vi "ArrayTransformations.vi"(10 "?":T1=enum."Transpose", 11 "Input":u32[][](array[numeric])) -> (3 "Transformed Array":u32[][](array[numeric]))   [LabVIEW 2017]
uses:
  Transformation Mode.ctl
panel:
  # "This VI shows how to apply all simple symmetry operations to a 2D array.\n\nChristian Altenbach, altenbach@gmail.com"
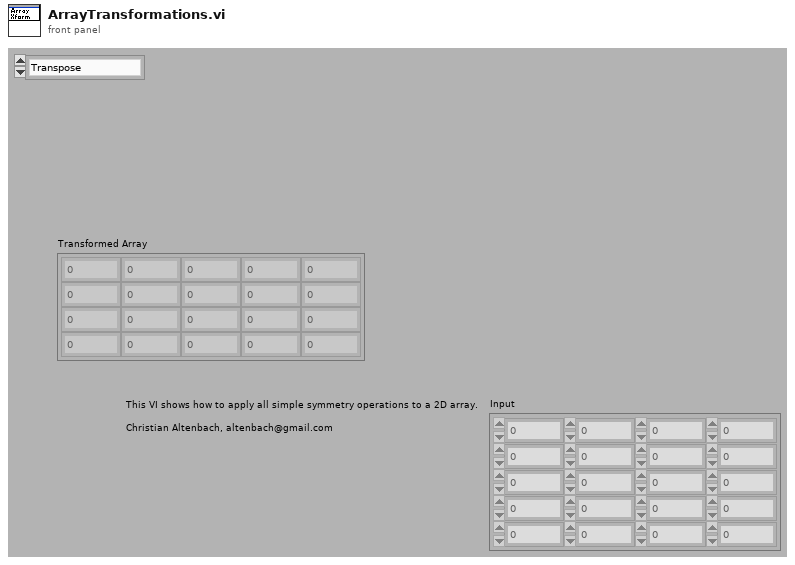
[diagram p1: front panel]
types:
  T1 = typedef "Transformation Mode.ctl" = enum16{"None", "Transpose", "Vertical Flip", "Horizontal Flip", "Rotate 90", "Rotate 270", "Rotate 180", "Diagonal Flip"}
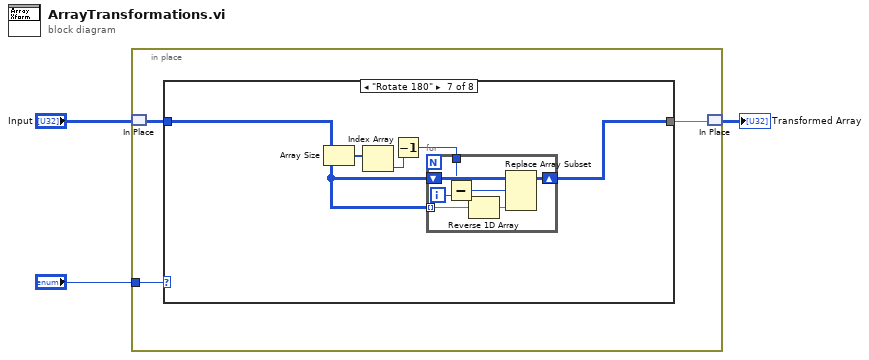
[diagram p0: block diagram]
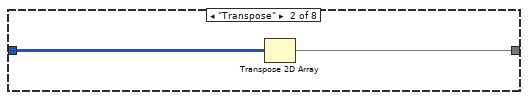
[diagram p3: hidden frame]
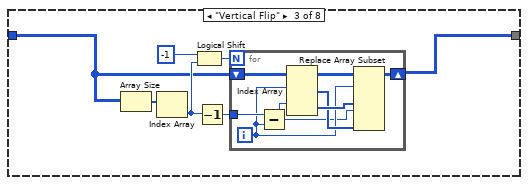
[diagram p4: hidden frame]
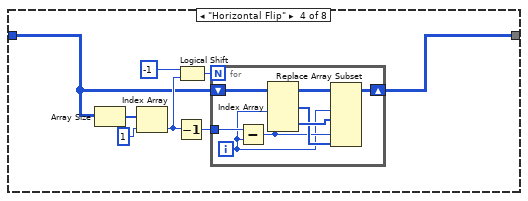
[diagram p5: hidden frame]
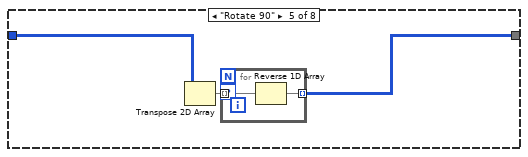
[diagram p6: hidden frame]
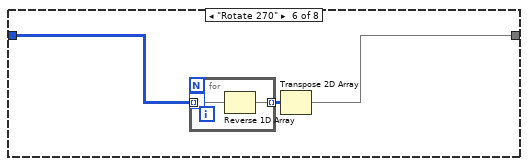
[diagram p7: hidden frame]
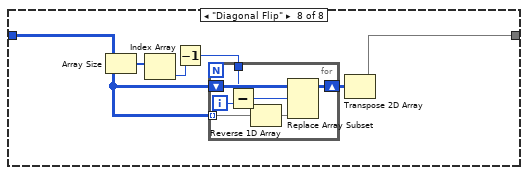
[diagram p8: hidden frame]
diagram:
  n1 = in-place {
    in-place-border: "?" -> [w6]
    n2 = in-place-match #1("Input") -> (w5:u32[][])
    n3 = case shown="\"Rotate 180\"" w6 {
      tunnel: w5 -> [w7 w9 w11 w25 w40 w45 w50 w62]
      tunnel: [w7 w8 w10 w24 w39 w44 w49 w61] -> w4
      frame "None", Default {
      }
      frame "Transpose" {
        n4 = Transpose 2D Array(2D array=w9) -> (transposed array=w8:u32[][])
      }
      frame "Vertical Flip" {
        n5 = Array Size(array=w11) -> (size(s)=w12:i32[])
        n6 = Index Array(array=w12) -> (element=w14:i32)  [unwired: 1 in]
        n7 = Logical Shift(y=i8 -1, x=w14) -> (x << y=w13:i32)
        n8 = Decrement(x=w14) -> (x-1=w16:i32)
        n9 = for {
          N: w13 -> [_]
          shift-right: [w23] -> w10
          shift-left: w11 -> [w22]
          tunnel: w16 -> [w19]
          i -> [w18]
          n10 = Subtract(x=w19, y=w18) -> (x-y=w17:i32)
          n11 = Index Array(array=w22, index (row) #1=w18, index (row) #2=w17) -> (element #1=w20:u32[], element #2=w21:u32[])  [unwired: 2 in]
          n12 = Replace Array Subset(array=w22, new element #1=w21, index (row) #1=w18, new element #2=w20, index (row) #2=w17) -> (w23:u32[][])  [unwired: 2 in]
        }
      }
      frame "Horizontal Flip" {
        n13 = Array Size(array=w25) -> (size(s)=w30:i32[])
        n14 = Index Array(array=w30, index=1) -> (element=w28:i32)
        n15 = Decrement(x=w28) -> (x-1=w26:i32)
        n16 = Logical Shift(y=i8 -1, x=w28) -> (x << y=w29:i32)
        n17 = for {
          N: w29 -> [_]
          shift-right: [w38] -> w24
          shift-left: w25 -> [w37]
          tunnel: w26 -> [w34]
          i -> [w32]
          n18 = Subtract(x=w34, y=w32) -> (x-y=w33:i32)
          n19 = Index Array(array=w37, index (col) #1=w32, index (col) #2=w33) -> (element #1=w35:u32[], element #2=w36:u32[])  [unwired: 2 in]
          n20 = Replace Array Subset(array=w37, new element #1=w36, index (col) #1=w32, new element #2=w35, index (col) #2=w33) -> (w38:u32[][])  [unwired: 2 in]
        }
      }
      frame "Rotate 90" {
        n21 = Transpose 2D Array(2D array=w40) -> (transposed array=w41:u32[][])
        n22 = for {
          tunnel: w41 -> [w43] mode=indexing
          tunnel: [w42] -> w39 mode=indexing
          workers-P: _ -> [_]
          n23 = Reverse 1D Array(array=w43) -> (reversed array=w42:u32[])
        }
      }
      frame "Rotate 270" {
        n24 = for {
          tunnel: w45 -> [w48] mode=indexing
          tunnel: [w47] -> w46 mode=indexing
          workers-P: _ -> [_]
          n25 = Reverse 1D Array(array=w48) -> (reversed array=w47:u32[])
        }
        n26 = Transpose 2D Array(2D array=w46) -> (transposed array=w44:u32[][])
      }
      frame "Rotate 180" {
        n27 = Array Size(array=w50) -> (size(s)=w51:i32[])
        n28 = Index Array(array=w51) -> (element=w53:i32)  [unwired: 1 in]
        n29 = Decrement(x=w53) -> (x-1=w52:i32)
        n30 = for {
          shift-right: [w60] -> w49
          shift-left: w50 -> [w59]
          tunnel: w52 -> [w57]
          tunnel: w50 -> [w54] mode=indexing
          i -> [w58]
          n31 = Subtract(x=w57, y=w58) -> (x-y=w56:i32)
          n32 = Reverse 1D Array(array=w54) -> (reversed array=w55:u32[])
          n33 = Replace Array Subset(array=w59, new element=w55, index (row)=w56) -> (w60:u32[][])  [unwired: 1 in]
        }
      }
      frame "Diagonal Flip" {
        n34 = Array Size(array=w62) -> (size(s)=w65:i32[])
        n35 = Index Array(array=w65) -> (element=w63:i32)  [unwired: 1 in]
        n36 = Decrement(x=w63) -> (x-1=w64:i32)
        n37 = for {
          shift-right: [w73] -> w66
          shift-left: w62 -> [w72]
          tunnel: w64 -> [w70]
          tunnel: w62 -> [w67] mode=indexing
          i -> [w71]
          n38 = Subtract(x=w70, y=w71) -> (x-y=w69:i32)
          n39 = Reverse 1D Array(array=w67) -> (reversed array=w68:u32[])
          n40 = Replace Array Subset(array=w72, new element=w68, index (row)=w69) -> (w73:u32[][])  [unwired: 1 in]
        }
        n41 = Transpose 2D Array(2D array=w66) -> (transposed array=w61:u32[][])
      }
    }
    n42 = in-place-match #1(w4) -> (→"Transformed Array":u32[][])
  }
